vi "GUI-Visibility-All FP Ctrl & Indi On-Off.vi"(0 "All Object Ref":refnum<vi>[](array[refnum]), 2 "Label In":string, 5 "All Object Label":string[](array[string]), 13 "Visible":bool) -> (4 "Ctl Refnum":refnum<vi>, 6 "Refnum Ok?":bool, 15 "error out":errorcluster)   [LabVIEW 2024]
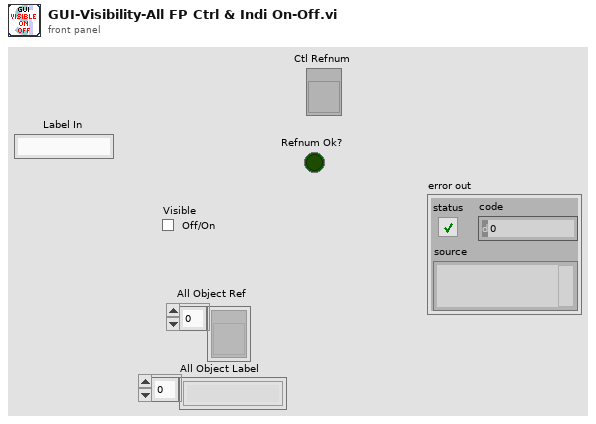
[diagram p1: front panel]
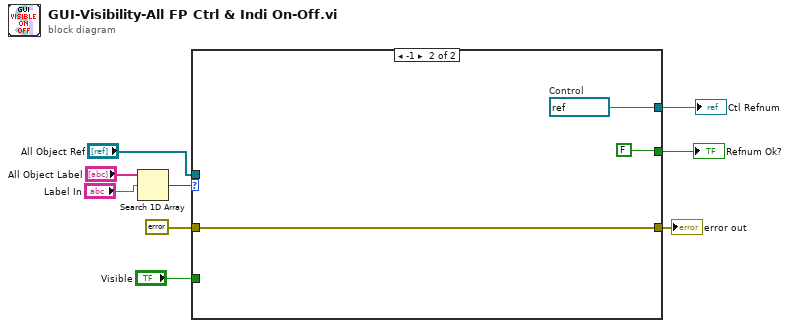
[diagram p0: block diagram]
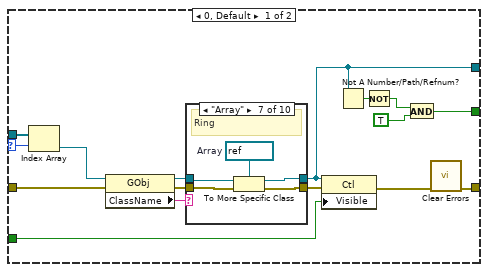
[diagram p2: hidden frame]
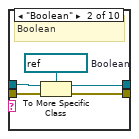
[diagram p4: hidden frame]
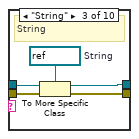
[diagram p5: hidden frame]
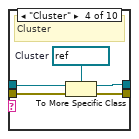
[diagram p6: hidden frame]
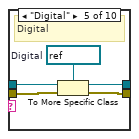
[diagram p7: hidden frame]
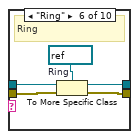
[diagram p8: hidden frame]
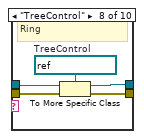
[diagram p9: hidden frame]
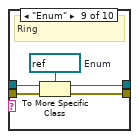
[diagram p10: hidden frame]
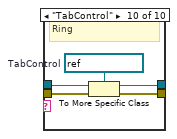
[diagram p11: hidden frame]
diagram:
  n1 = Search 1D Array(1D array="All Object Label", element="Label In") -> (index of element=w5:i32)  [unwired: 1 in]
  n2 = case shown="-1" w5 {
    selector: w5 -> [w19 _]
    tunnel: [w22 w74] -> w8
    tunnel: "Visible" -> [w21 _]
    tunnel: errorcluster {"status"=FALSE, "code"=0, "source"=""} ("error in (no error)") -> [w20 w74]
    tunnel: "All Object Ref" -> [w18 _]
    tunnel: [w11 w73] -> w2
    tunnel: [w10 FALSE] -> w1
    frame 0, Default {
      n3 = Index Array(array=w18, index=w19) -> (element=w17:refnum<vi>)
      n4 = property class="GObj"(reference=w17, error in=w20) -> (reference out=w15:refnum<vi>, error out=w24:errorcluster, "ClassName"=w25:string)
      n5 = case shown="\"Array\"" w25 {
        tunnel: w15 -> [_ w31 w36 w41 w46 w51 w56 w61 w66 w71]
        tunnel: [_ w27 w34 w39 w43 w49 w54 w59 w64 w68] -> w11
        tunnel: w24 -> [w26 w29 w33 w38 w44 w48 w53 w58 w63 w69]
        tunnel: [w26 w28 w32 w37 w42 w47 w52 w57 w62 w67] -> w23
        frame Default {
        }
        frame "Boolean" {
          w30 = refnum<vi> refnum  # Boolean
          # "Boolean"
          n6 = To More Specific Class(target class=w30, reference=w31, error in=w29) -> (specific class reference=w27:refnum<vi>, error out=w28:errorcluster)
        }
        frame "String" {
          w35 = refnum<vi> refnum  # String
          # "String"
          n7 = To More Specific Class(target class=w35, reference=w36, error in=w33) -> (specific class reference=w34:refnum<vi>, error out=w32:errorcluster)
        }
        frame "Cluster" {
          w40 = refnum<vi> refnum  # Cluster
          # "Cluster"
          n8 = To More Specific Class(target class=w40, reference=w41, error in=w38) -> (specific class reference=w39:refnum<vi>, error out=w37:errorcluster)
        }
        frame "Digital" {
          w45 = refnum<vi> refnum  # Digital
          # "Digital"
          n9 = To More Specific Class(target class=w45, reference=w46, error in=w44) -> (specific class reference=w43:refnum<vi>, error out=w42:errorcluster)
        }
        frame "Ring" {
          w50 = refnum<vi> refnum  # Ring
          # "Ring"
          n10 = To More Specific Class(target class=w50, reference=w51, error in=w48) -> (specific class reference=w49:refnum<vi>, error out=w47:errorcluster)
        }
        frame "Array" {
          w55 = refnum<vi> refnum  # Array
          # "Ring"
          n11 = To More Specific Class(target class=w55, reference=w56, error in=w53) -> (specific class reference=w54:refnum<vi>, error out=w52:errorcluster)
        }
        frame "TreeControl" {
          w60 = refnum<vi> refnum  # TreeControl
          # "Ring"
          n12 = To More Specific Class(target class=w60, reference=w61, error in=w58) -> (specific class reference=w59:refnum<vi>, error out=w57:errorcluster)
        }
        frame "Enum" {
          w65 = refnum<vi> refnum  # Enum
          # "Ring"
          n13 = To More Specific Class(target class=w65, reference=w66, error in=w63) -> (specific class reference=w64:refnum<vi>, error out=w62:errorcluster)
        }
        frame "TabControl" {
          w70 = refnum<vi> refnum  # TabControl
          # "Ring"
          n14 = To More Specific Class(target class=w70, reference=w71, error in=w69) -> (specific class reference=w68:refnum<vi>, error out=w67:errorcluster)
        }
      }
      n15 = property class="Ctl"(reference=w11, error in=w23, "Visible"=w21) -> (error out=w16:errorcluster)  [unwired: 1 out]
      n16 = Not A Number/Path/Refnum?(number/path/refnum=w11) -> (NaN/Path/Refnum?=w14:bool)
      n17 = Not(x=w14) -> (.not. x?=w13:bool)
      n18 = And(x=w13, y=TRUE) -> (x .and. y?=w10:bool)
      n19 = call <vilib>:"Clear Errors.vi"("error in (no error)"=w16) -> ("error out"=w22:errorcluster)  [unwired: 5 in, 1 out]
    }
    frame -1 {
      w73 = refnum<vi> refnum  # Control
    }
  }
  "error out" <- w8
  "Ctl Refnum" <- w2
  "Refnum Ok?" <- w1
